vi "Sweep_Test_logging.vi"() -> ()   [LabVIEW 2026]
uses:
  <vilib>/Utility/file.llb/Write Delimited Spreadsheet (DBL).vi
panel:
  out "Last Saved To":string
  in  "Serial Number":string
  out "Fail Count":dbl
  out "Overall PASS":bool
  in  "Gain Max (dB)":dbl
  in  "Gain Min (dB)":dbl
  out "Gain vs Frequency":cluster{dbl[], dbl[]}(graph)
  in  "Step (MHz)":dbl
  in  "Stop (MHz)":dbl
  in  "Start (MHz)":dbl
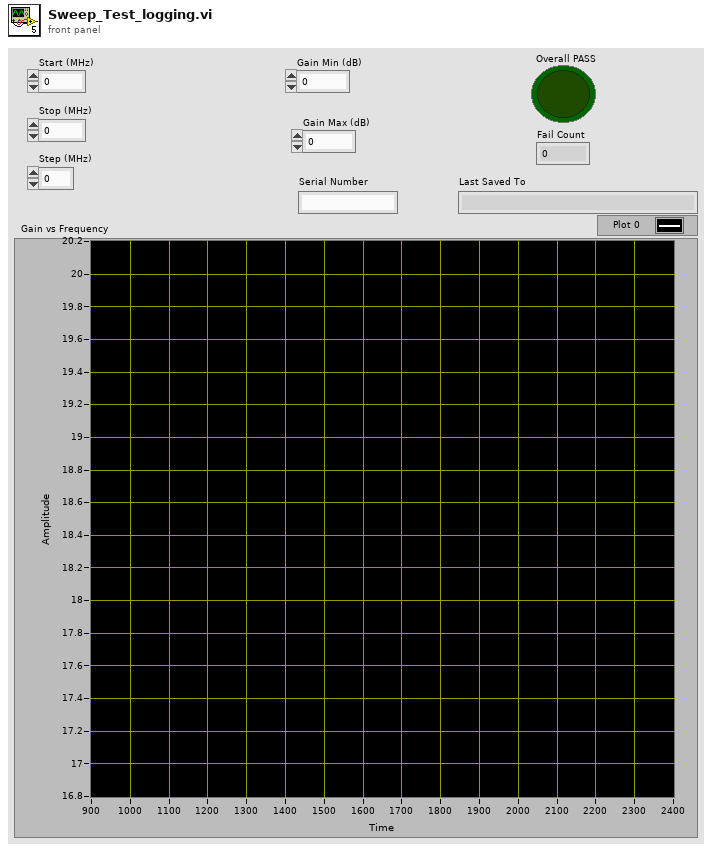
[diagram p1: front panel]
types:
  T1 = enum16{"open", "replace", "create", "open or create", "replace or create", "replace or create with confirmation"}
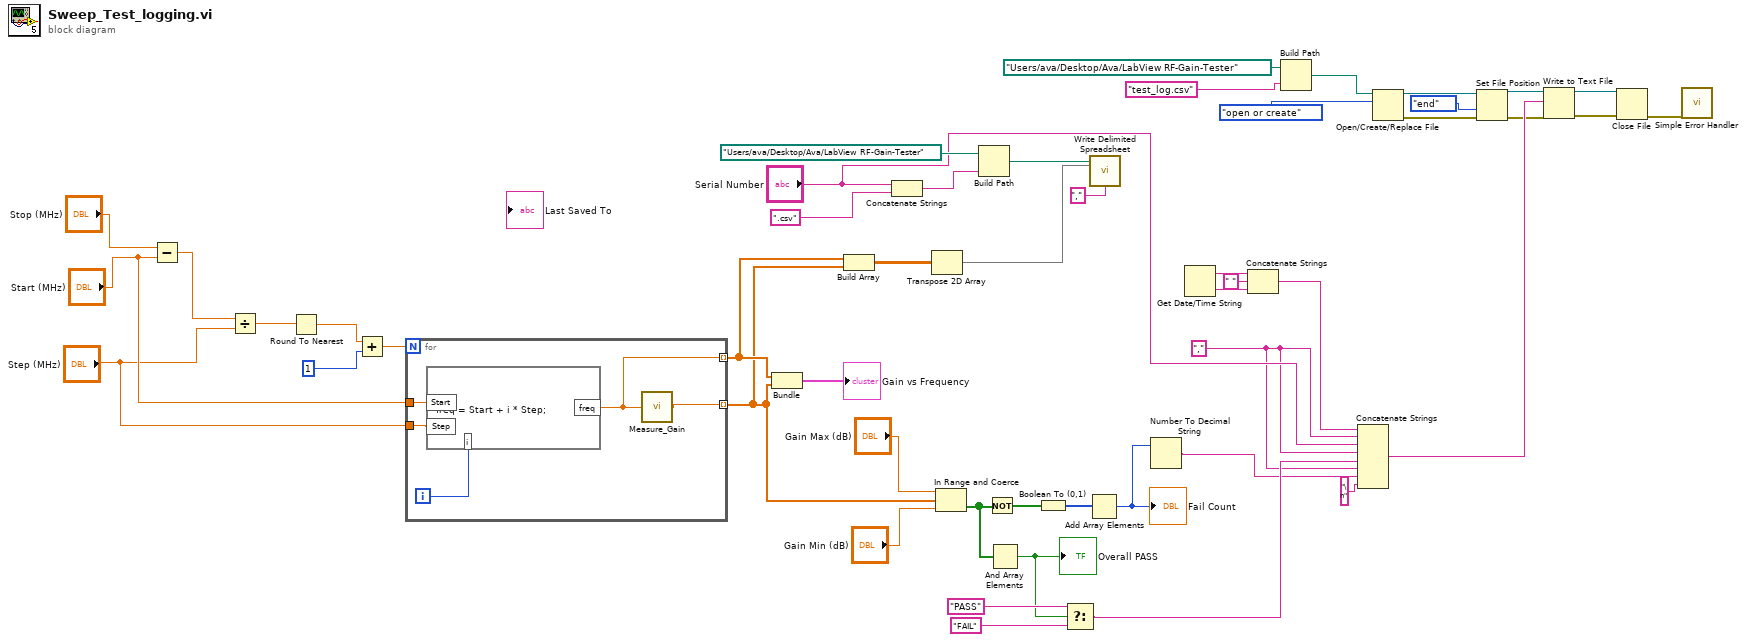
[diagram p0: block diagram]
diagram:
  w16 = "," ("string")
  n1 = Subtract(x="Stop (MHz)", y="Start (MHz)") -> (x-y=w48:dbl)
  n2 = Divide(x=w48, y="Step (MHz)") -> (x/y=w47:dbl)
  n3 = Round To Nearest(number=w47) -> (nearest integer value=w46:dbl)
  n4 = Add(x=w46, y=1) -> (x+y=w44:dbl)
  n5 = for {
    N: w44 -> [_]
    tunnel: "Start (MHz)" -> [w54]
    tunnel: "Step (MHz)" -> [w53]
    tunnel: [w51] -> w34 mode=indexing
    tunnel: [w50] -> w35 mode=indexing
    i -> [w52]
    n6 = formula code="freq = Start + i * Step;"("Start"=w54, "Step"=w53, "i"=w52) -> ("freq"=w50:dbl)
    n7 = call "Measure_Gain.vi"("Frequency (MHz)"=w50) -> ("Gain (dB)"=w51:dbl)
  }
  n8 = Bundle(w35, w34) -> (→"Gain vs Frequency":cluster{dbl[], dbl[]})  [unwired: 1 in]
  n9 = Build Array(w35, w34) -> (w33:dbl[][])
  n10 = Concatenate Strings("Serial Number", ".csv") -> (w30:string)
  n11 = Transpose 2D Array(2D array=w33) -> (transposed array=w29:dbl[][])
  n12 = In Range and Coerce(upper limit="Gain Max (dB)", x=w34, lower limit="Gain Min (dB)") -> (In Range?=w36:bool[])  [unwired: 1 out]
  n13 = Build Path(base path=path "/Users/ava/Desktop/Ava/LabView RF-Gain-Tester", name or relative path=w30) -> (appended path=w28:path)
  n14 = Not(x=w36) -> (.not. x?=w38:bool[])
  n15 = And Array Elements(Boolean array=w36) -> (logical AND=w21:bool)
  "Overall PASS" <- w21
  n16 = Boolean To (0,1)(Boolean=w38) -> (0, 1=w37:i16[])
  n17 = Select(t="PASS", s=w21, f="FAIL") -> (s? t:f=w17:string)
  n18 = Add Array Elements(numeric array=w37) -> (sum=w20:i16)
  "Fail Count" <- w20
  n19 = call-poly <vilib>:"Write Delimited Spreadsheet.vi"("file path (dialog if empty)"=w28, "2D data"=w29, "delimiter (\\t)"="," ("delimiter (\\t)")) -> ()  [unwired: 11 in, 2 out]
  n20 = Number To Decimal String(number=w20) -> (decimal integer string=w15:string)  [unwired: 1 in]
  n21 = Get Date/Time String() -> (date string=w26:string, time string=w25:string)  [unwired: 3 in]
  n22 = Concatenate Strings(w26, " " ("string"), w25) -> (w19:string)
  n23 = Build Path(base path=path "/Users/ava/Desktop/Ava/LabView RF-Gain-Tester", name or relative path="test_log.csv") -> (appended path=w12:path)
  n24 = Concatenate Strings(w19, w16, "Serial Number", w16, w17, w16, w15, "\n" ("string")) -> (w7:string)
  n25 = Open/Create/Replace File(file path (use dialog)=w12, operation (0:open)=T1."open or create") -> (refnum out=w10:refnum<file>, error out=w5:errorcluster)  [unwired: 4 in, 1 out]
  n26 = Set File Position(refnum=w10, from (0:start)=enum16{"start", "end", "current"}."end", error in=w5) -> (refnum out=w8:refnum<file>, error out=w4:errorcluster)  [unwired: 1 in]
  n27 = Write to Text File(file (use dialog)=w8, text=w7, error in=w4) -> (refnum out=w6:refnum<file>, error out=w3:errorcluster)  [unwired: 1 in, 1 out]
  n28 = Close File(refnum=w6, error in=w3) -> (error out=w2:errorcluster)  [unwired: 1 out]
  n29 = call <vilib>:"Simple Error Handler.vi"("error in (no error)"=w2) -> ()  [unwired: 4 in, 5 out]
